vi "Atheros MEM COMMIT.vi"(0 "_hResourceContext":u32, 5 "CommitMemPara":T1, 11 "error in (no error)":errorcluster) -> (4 "_hResourceContext out":u32, 8 "function return":bool, 15 "error out":errorcluster)   [LabVIEW 2013, in "QCAWLAN_DLL.lvlib"]
doc: "QCA_DLL_Export bool Atheros_MEM_COMMIT(HANDLE _hResourceContext, unsigned char iTemplateNum, unsigned char iWriteOption, unsigned long iMemSize, unsigned char iCompress, unsigned char iOverwrite, int* iSectionMask);"
uses:
  QCAWLAN_DLL.lvlib
  QCAWLAN_DLL.dll
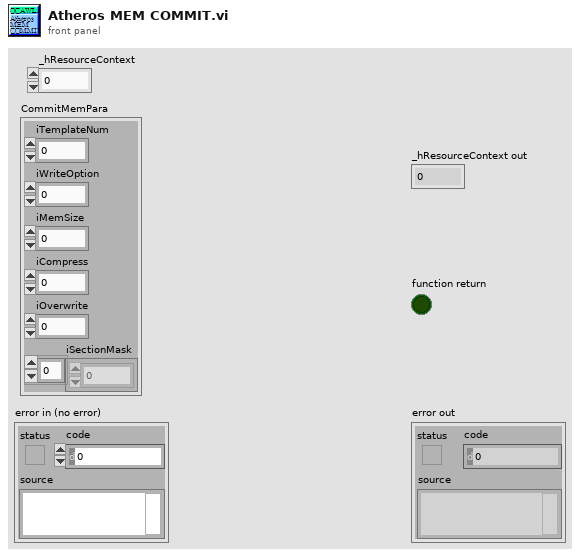
[diagram p1: front panel]
types:
  T1 = cluster{"iTemplateNum":u8, "iWriteOption":u8, "iMemSize":u32, "iCompress":u8, "iOverwrite":u8, "iSectionMask":i32[]}
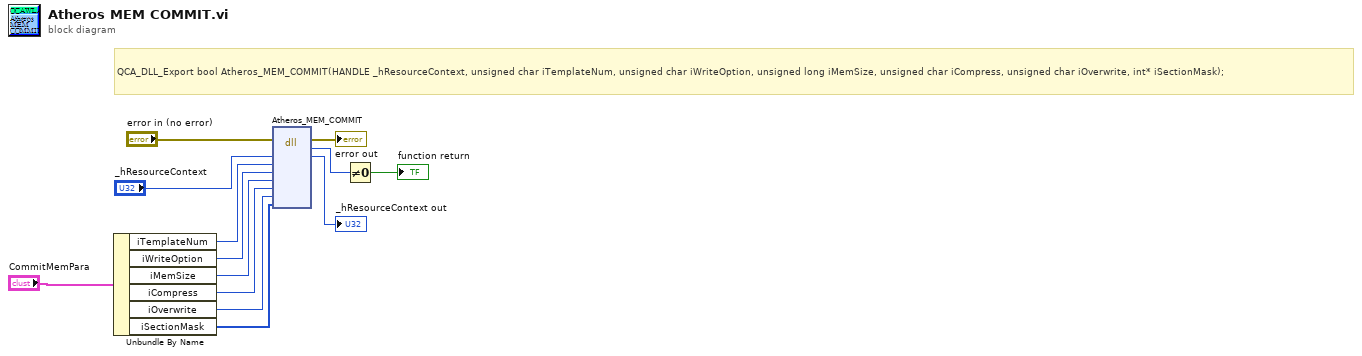
[diagram p0: block diagram]
diagram:
  # "QCA_DLL_Export bool Atheros_MEM_COMMIT(HANDLE _hResourceContext, unsigned char iTemplateNum, unsigned char iWriteOption, unsigned long iMemSize, unsigned char iCompress, unsigned char iOverwrite, int* iSectionMask);"
  n1 = Unbundle By Name("CommitMemPara") -> ("iTemplateNum"=w6:u8, "iWriteOption"=w5:u8, "iMemSize"=w4:u32, "iCompress"=w3:u8, "iOverwrite"=w2:u8, "iSectionMask"=w1:i32[])
  n2 = dll-call lib="C:/Connectivity Client - MIMO/PlugIn/QCAWLAN_DLL.*" fn="Atheros_MEM_COMMIT"(error in="error in (no error)", "_hResourceContext"="_hResourceContext", "iTemplateNum"=w6, "iWriteOption"=w5, "iMemSize"=w4, "iCompress"=w3, "iOverwrite"=w2, "iSectionMask"=w1) -> (error out=→"error out":errorcluster, "return type"=w12:u8, "_hResourceContext"=→"_hResourceContext out":u32)  [unwired: 8 in, 1 out]
  n3 = Not Equal To 0?(x=w12) -> (x != 0?=→"function return":bool)
